vi "functional global counter 2.vi"() -> ()   [LabVIEW 2009]
uses:
  Functional Global Command.ctl
panel:
  out "Compte 2":i32
  out "total cumulatif":i32
  out "Compte total":i32
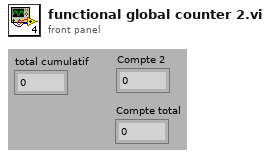
[diagram p1: front panel]
types:
  T1 = typedef "Functional Global Command.ctl" = enum16{"Réinitialiser", "Incrémenter", "Obtenir le compte"}
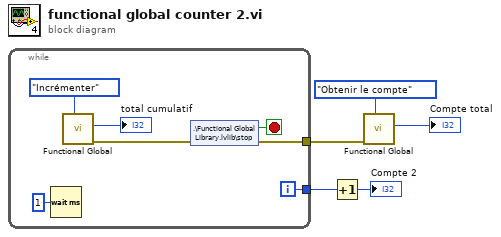
[diagram p0: block diagram]
diagram:
  n1 = while "Boucle While" {
    tunnel: [w12] -> w5
    tunnel: [w11] -> w3
    i -> [w12]
    stop <- w6 stop-if-true
    n2 = Wait (ms) ("Attendre (ms)")(milliseconds to wait=u32 1) -> ()  [unwired: 1 out]
    n3 = call "Functional Global.vi"("Commande"=Functional_Global_Command."Incrémenter" ("Command")) -> ("sortie d'erreur"=w8:errorcluster, "Compte"=→"total cumulatif":i32)  [unwired: 9 in]
    n4 = shared-variable ".\\Functional Global Library.lvlib\\stop"(error in=w8) -> (w6:bool, error out=w11:errorcluster)
  }
  n5 = Increment ("Incrémenter")(x=w5) -> (x+1=→"Compte 2":i32)
  n6 = call "Functional Global.vi"("Commande"=Functional_Global_Command."Obtenir le compte" ("Command"), "entrée d'erreur (pas d'erreur)"=w3) -> ("Compte"=→"Compte total":i32)  [unwired: 8 in, 1 out]
